vi "Apply Manipulation.vi"(8 "error in (no error)":errorcluster, 10 "Data in":dbl[][](array[numeric]), 11 "Abstract Data Manipulator in":refnum<class "Abstract Data Manipulator.lvclass">) -> (0 "error out":errorcluster, 2 "Data out":dbl[][](array[numeric]), 3 "Abstract Data Manipulator out":refnum<class "Abstract Data Manipulator.lvclass">)   [LabVIEW 2016, in "Abstract Data Manipulator.lvclass"]
uses:
  Abstract Data Manipulator.lvclass
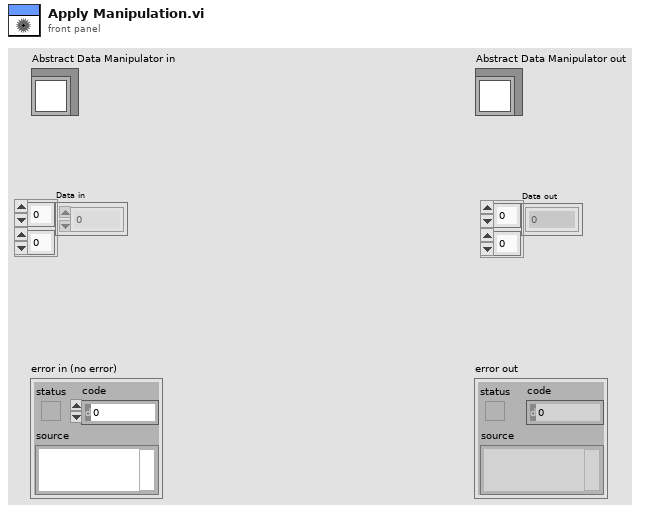
[diagram p1: front panel]
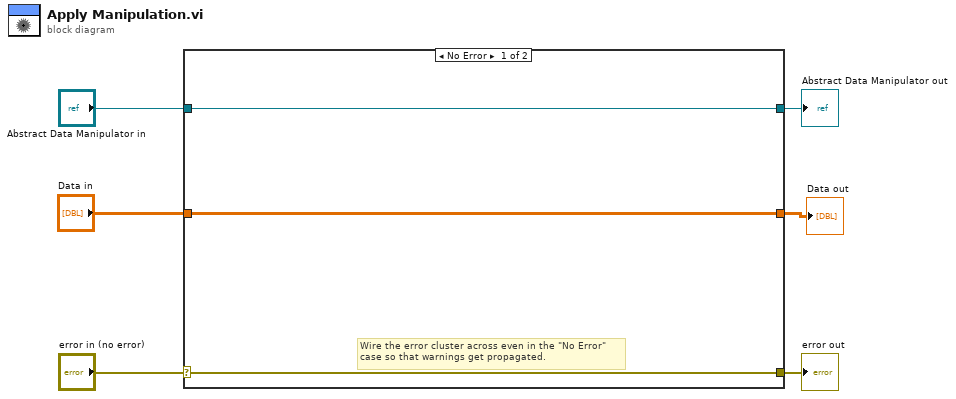
[diagram p0: block diagram]
diagram:
  n1 = case shown="No Error" "error in (no error)" {
    selector: "error in (no error)" -> [w8 w12]
    tunnel: [w8 w12] -> w5
    tunnel: [w9 w11] -> w3
    tunnel: "Abstract Data Manipulator in" -> [w9 w11]
    tunnel: [w7 w10] -> w2
    tunnel: "Data in" -> [w7 w10]
    frame No Error {
      # "Wire the error cluster across even in the \"No Error\"\ncase so that warnings get propagated."
    }
    frame Error {
    }
  }
  "error out" <- w5
  "Abstract Data Manipulator out" <- w3
  "Data out" <- w2
